vi "Initialise.vi"(8 "error in (no error)":errorcluster, 10 "Instrument Ref":string, 11 "Keysight 5700C in":refnum<class "Keysight 5700C.lvclass">) -> (0 "error out":errorcluster, 3 "Keysight 5700C out":refnum<class "Keysight 5700C.lvclass">)   [LabVIEW 2021, in "Concrete.lvlib" / "Keysight 5700C.lvclass"]
uses:
  Keysight 5700C.lvclass
  Keysight 5700C.lvclass/Keysight 5700C.ctl
  Harware Abstraction/AnalogIO/Power Supply.lvclass
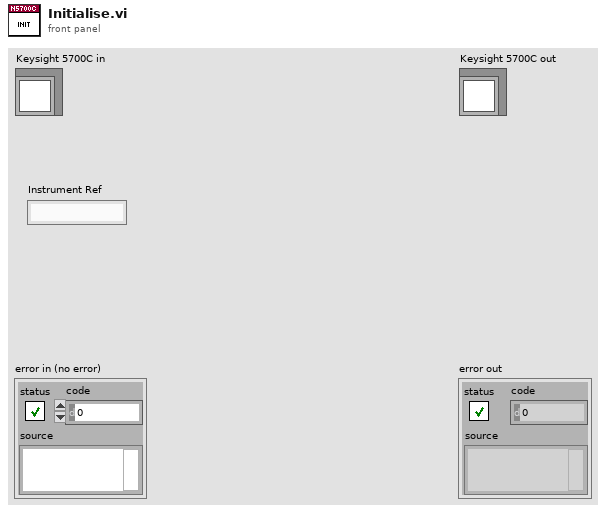
[diagram p1: front panel]
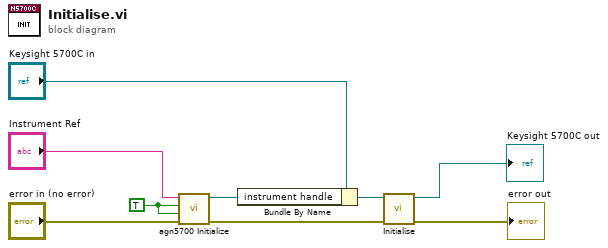
[diagram p0: block diagram]
diagram:
  w1 = TRUE ("id query (Yes)")
  n1 = call <instrlib>:"agn5700 Initialize.vi"("error in (no error)"="error in (no error)", "reset device (Yes)"=w1, "id query (Yes)"=w1, "resource name"="Instrument Ref") -> ("error out"=w4:errorcluster, "instrument handle out"=w2:refnum<k15>)  [unwired: 6 out]
  n2 = Bundle By Name(cluster="Keysight 5700C in", "instrument handle"=w2) -> (w6:refnum<class "Keysight 5700C.lvclass">)
  n3 = call-parent "Initialise.vi"("error in (no error)"=w4, "Instrument in"=w6) -> ("error out"=→"error out":errorcluster, "Instrument out"=→"Keysight 5700C out":refnum<class "Keysight 5700C.lvclass">)  [unwired: 8 in]
